vi "Camera Manager Simulation Image Source.vi"(8 "error in (no error)":errorcluster, 11 "chrArrImageSource":string) -> (0 "error out":errorcluster, 3 "chrArrImageSource out":string)   [LabVIEW 2017, in "PlayNitrideCameraComponet1010_4.lvlib"]
doc: "__declspec(dllexport) void CameraManager_SimulationImageSource(char* chrArrImageSource);"
uses:
  <userlib>/PlayNitrideCameraComponet1010_4/PlayNitrideCameraComponet1010_4.lvlib
  <userlib>/PlayNitrideCameraComponet1010_4/PlayNitrideCameraComponet.dll
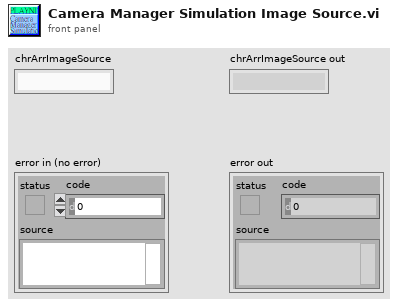
[diagram p1: front panel]
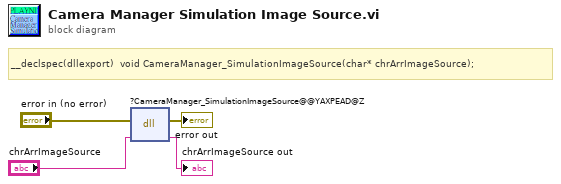
[diagram p0: block diagram]
diagram:
  # "__declspec(dllexport)  void CameraManager_SimulationImageSource(char* chrArrImageSource);"
  n1 = dll-call lib="C:/Program Files/National Instruments/LabVIEW 2017/user.lib/PlayNitrideCameraComponet1010_4/PlayNitrideCameraComponet.*" fn="?CameraManager_SimulationImageSource@@YAXPEAD@Z"(error in="error in (no error)", "chrArrImageSource"="chrArrImageSource") -> (error out=→"error out":errorcluster, "chrArrImageSource"=→"chrArrImageSource out":string)  [unwired: 3 in, 1 out]
